vi "dscGetStatus.vi"(8 "error in":errorcluster, 11 "board":i16) -> (0 "error out":errorcluster, 2 "status":T1 {"analog" items=["FALSE", "TRUE"]}, 3 "boardOut":i16)   [LabVIEW 2011, in "Diamond Universal Driver.lvlib"]
uses:
  Diamond Universal Driver.lvlib
  DSCS.ctl
  Controls/dscBool.ctl
  Controls/error codes.ctl
  Instruments/WL OPC/Support/dlls/dscud.dll
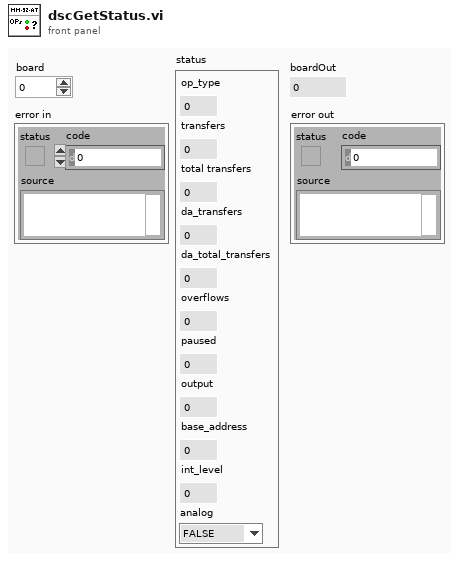
[diagram p1: front panel]
types:
  T1 = typedef "Diamond Universal Driver.lvlib/DSCS.ctl" = cluster{"op_type":u8, "transfers":u32, "total transfers":u32, "da_transfers":u32, "da_total_transfers":u32, "overflows":u32, "paused":u8, "output":u8, "base_address":u16, "int_level":u8, "analog":T2}
  T2 = typedef "dscBool.ctl" = i32
  T3 = typedef "Diamond Universal Driver.lvlib/error codes.ctl" = enum8{"DE_NONE", "DE_HW_FAILURE", "DE_SW_FAILURE", "DE_HW_NOT_SUPPORTED", "DE_SW_NOT_SUPPORTED", "DE_INVALID_PARM", "DE_ALTERNATE_IN_PROGRESS", "DE_NONE_IN_PROGRESS", "DE_BUFFER_ROLLOVER", "DE_INVALID_ERROR_CODE", "DE_ALREADY_PAUSED", "DE_OVERFLOW", "DE_INVALID_FUNC", "DE_DSCUDH_INVALID", "DE_INVALID_BOARD", "DE_BOARD_LIMIT_REACHED", "DE_BOARD_BUSY", "DE_INVALID_WINDRVR_HANDLE", "DE_INVALID_WINDRVR_VERSION", "DE_BAD_WINDRVR_BOARD_INIT", "DE_OPERATION_TIMED_OUT", "DE_INVALID_WINDRVR_KP", "DE_THREAD_FAILURE"}
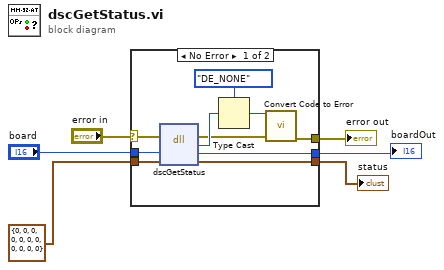
[diagram p0: block diagram]
diagram:
  n1 = case shown="No Error" "error in" {
    selector: "error in" -> [w16 w19]
    tunnel: T1 {"op_type"=0, "transfers"=0, "total transfers"=0, "da_transfers"=0, "da_total_transfers"=0, "overflows"=0, "paused"=0, "output"=0, "base_address"=0, "int_level"=0, "analog"=0} ("dscs") -> [w15 w18]
    tunnel: "board" -> [w14 w17]
    tunnel: [w9 w19] -> w4
    tunnel: [w8 w18] -> w3
    tunnel: [w7 w17] -> w2
    frame No Error {
      n2 = dll-call lib="C:/Users/mrichardson/Documents/Web Based Version Control SW/Instruments/WL OPC/Support/dlls/dscud.dll" fn="dscGetStatus"(error in=w16, "board"=w14, "status"=w15) -> (error out=w11:errorcluster, "error"=w12:u8, "board"=w7:i16, "status"=w8:T1)  [unwired: 2 in, 1 out]
      n3 = Type Cast(type=error_codes."DE_NONE" ("error codes"), x=w12) -> (*(type *) &x=w10:T3)
      n4 = call "Convert Code to Error.vi"("error in"=w11, "error codes"=w10) -> ("error out"=w9:errorcluster)  [unwired: 9 in]
    }
    frame Error {
    }
  }
  "error out" <- w4
  "status" <- w3
  "boardOut" <- w2
